vi "探头静音与恢复切换.vi"(7 "VISA资源名称":refnum<visa-resource-name>, 8 "探头地址":u8, 9 "限值1":dbl, 11 "切换至方式":T1) -> (2 "切换成功？":bool)   [LabVIEW 2017]
panel:
  out "读取缓冲区":string
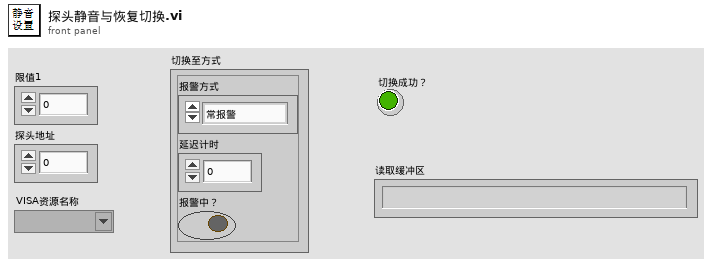
[diagram p1: front panel]
types:
  T1 = cluster{"报警方式":enum16{"常报警", "自动静音", "手动静音"}, "延迟计时":u16, "报警中？":bool}
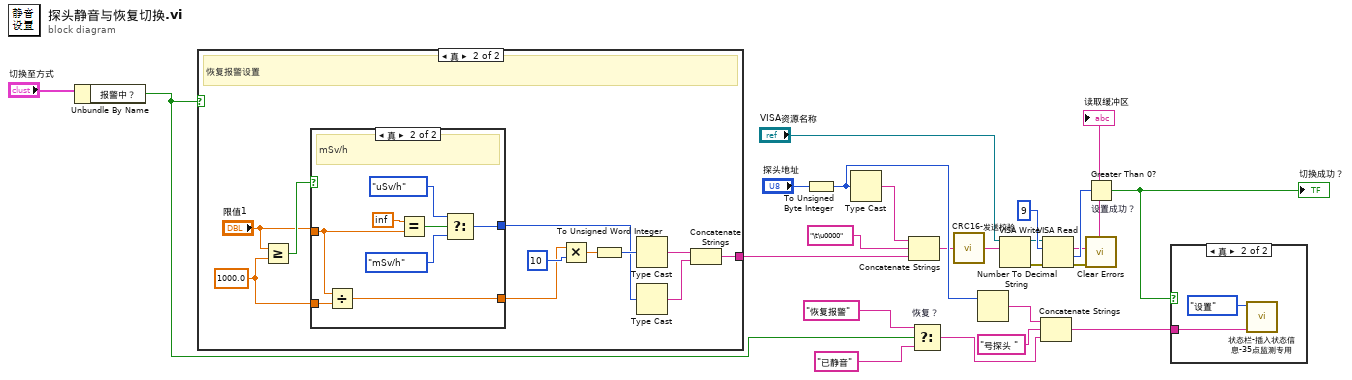
[diagram p0: block diagram]
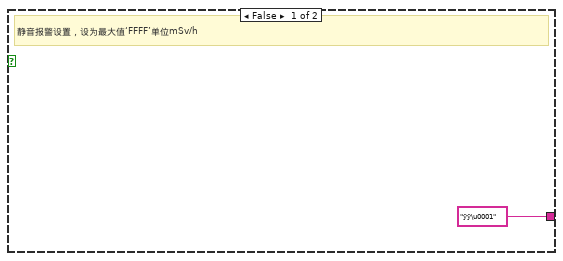
[diagram p3: hidden frame]
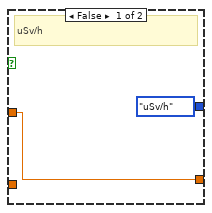
[diagram p4: hidden frame]
diagram:
  n1 = Unbundle By Name("切换至方式") -> ("报警中？"=w2:bool)
  n2 = case shown="真" w2 {
    tunnel: ["ÿÿ\u0001" w25] -> w4
    frame False {
      # "静音报警设置，设为最大值‘FFFF’单位mSv/h"
    }
    frame True {
      w33 = 1000.0 ("y")
      # "恢复报警设置"
      n3 = Greater Or Equal?(x="限值1", y=w33) -> (x >= y?=w35:bool)
      n4 = case shown="真" w35 {
        tunnel: "限值1" -> [w36 w43]
        tunnel: w33 -> [_ w45]
        tunnel: [w36 w44] -> w29
        tunnel: [enum8{"uSv/h", "mSv/h"}."uSv/h" ("单位1") w38] -> w28
        frame False {
          # "uSv/h"
        }
        frame True {
          # "mSv/h"
          n5 = Divide(x=w43, y=w45) -> (x/y=w44:dbl)
          n6 = Equal?(x=inf, y=w43) -> (x = y?=w41:bool)
          n7 = Select(t=enum8{"uSv/h", "mSv/h"}."uSv/h" ("单位1"), s=w41, f=enum8{"uSv/h", "mSv/h"}."mSv/h" ("单位1")) -> (s? t:f=w38:enum8{"uSv/h", "mSv/h"})
        }
      }
      n8 = Multiply(x=w29, y=10) -> (x*y=w31:dbl)
      n9 = To Unsigned Word Integer(number=w31) -> (unsigned 16bit integer=w32:u16)
      n10 = Type Cast(x=w32) -> (*(type *) &x=w27:string)  [unwired: 1 in]
      n11 = Type Cast(x=w28) -> (*(type *) &x=w26:string)  [unwired: 1 in]
      n12 = Concatenate Strings(w27, w26) -> (w25:string)
    }
  }
  n13 = To Unsigned Byte Integer(number="探头地址") -> (unsigned 8bit integer=w19:u8)
  n14 = Type Cast(x=w19) -> (*(type *) &x=w10:string)  [unwired: 1 in]
  n15 = Concatenate Strings(w10, "\t\u0000", w4) -> (w7:string)
  n16 = Select "恢复？"(t="恢复报警", s=w2, f="已静音") -> (s? t:f=w22:string)
  n17 = call "CRC16-发送校验.vi"("净数据"=w7) -> ("完整输出"=w9:string)
  n18 = Number To Decimal String(number=w19) -> (decimal integer string=w20:string)  [unwired: 1 in]
  n19 = VISA Write(VISA resource name="VISA资源名称", write buffer=w9) -> (VISA resource name out=w12:refnum<visa-resource-name>, error out=w11:errorcluster)  [unwired: 1 in, 1 out]
  n20 = Concatenate Strings(w20, "号探头 ", w22) -> (w23:string)
  n21 = VISA Read(VISA resource name=w12, byte count=u32 9 ("字节总数"), error in (no error)=w11) -> (read buffer=→"读取缓冲区":string, return count=w14:u32, error out=w15:errorcluster)  [unwired: 1 out]
  n22 = Greater Than 0? "设置成功？"(x=w14) -> (x > 0?=w16:bool)
  "切换成功？" <- w16
  n23 = call <vilib>:"Clear Errors.vi"("error in (no error)"=w15) -> ()  [unwired: 5 in, 2 out]
  n24 = case shown="真" w16 {
    tunnel: w23 -> [_ w46]
    frame False {
    }
    frame True {
      n25 = call "状态栏-插入状态信息-35点监测专用.vi"("消息内容"=w46, "状态类型"=enum16{"全部", "报警", "通信", "设置"}."设置") -> ()  [unwired: 10 in]
    }
  }
